vi "WorkorderHandler_Close.vi"(0 "reference":T1, 5 "error in (no error)":errorcluster) -> (19 "error out":errorcluster)   [LabVIEW 2011]
doc: "Closes a reference to a dqGOOP object. This should only be called to close additional references that were obtained by \"getObjectReference\" which looks up a named object and returns a unique refnum."
uses:
  DataStructures/WorkorderHandler_ObjectReference.ctl
  DataStructures/WorkorderHandler_ObjectData.ctl
panel:
  in  "queue (default)":refnum<queue>
  # "Copyright (C) 2004 DataAct Incorporated"
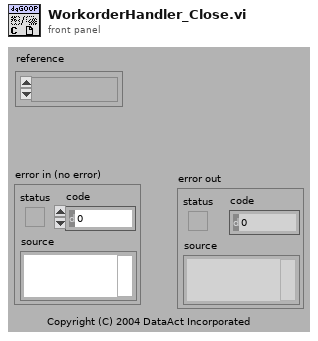
[diagram p1: front panel]
types:
  T1 = typedef "WorkorderHandler_ObjectReference.ctl" = refnum<k1>
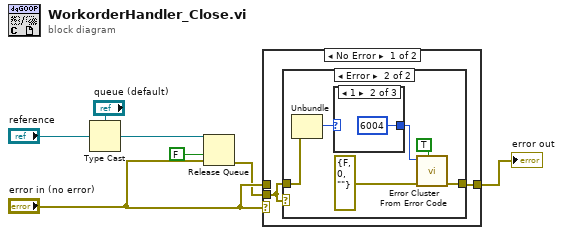
[diagram p0: block diagram]
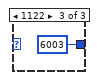
[diagram p4: hidden frame]
diagram:
  n1 = Type Cast(type="queue (default)", x="reference") -> (*(type *) &x=w5:refnum<queue>)
  n2 = Release Queue(queue=w5, force destroy? (F)=FALSE, error in (no error)="error in (no error)") -> (error out=w2:errorcluster)  [unwired: 2 out]
  n3 = case shown="No Error" "error in (no error)" {
    tunnel: [w8 w20] -> w1
    tunnel: "error in (no error)" -> [_ w20]
    tunnel: w2 -> [w9 _]
    frame No Error {
      n4 = case shown="Error" w9 {
        tunnel: [w10 w11] -> w8
        tunnel: w9 -> [w10 w16]
        frame No Error {
        }
        frame Error {
          n5 = Unbundle(w16) -> ("code"=w15:i32)  [unwired: 2 out]
          n6 = case shown="1" w15 {
            selector: w15 -> [w17 _ _]
            tunnel: [w17 6004 ("code") 6003 ("code")] -> w13
            frame Default {
            }
            frame 1 {
            }
            frame 1122 {
            }
          }
          n7 = call <vilib>:"Error Cluster From Error Code.vi"("show call chain? (False)"=TRUE, "error in (no error)"=errorcluster {"status"=FALSE, "code"=0, "source"=""} ("error out"), "error code (0)"=w13) -> ("error out"=w11:errorcluster)  [unwired: 6 out]
        }
      }
    }
    frame Error {
    }
  }
  "error out" <- w1
